vi "Do_channel_maths.vi"(4 "Output Index":i32, 5 "Channel Values In":string[][](array[string]), 6 "Channel Names":string[](array[string]), 7 "Maths Equation":string) -> (0 "Error String":string, 1 "Channel Values Out":string[][](array[string]))   [LabVIEW 2015]
uses:
  Data_plotting_vis/Results_plotter_Global.vi
  <vilib>/gmath/NI_Gmath.lvlib
panel:
  out "Generic Equation":string
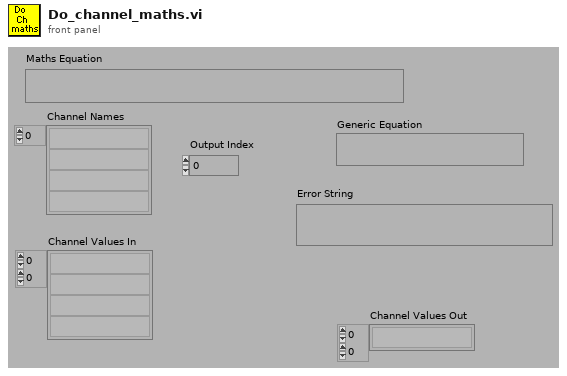
[diagram p1: front panel]
types:
  T1 = cluster{"Tables":i32[][], "Y Values":dbl[], "Variables input decode":i32[], i32[]}[]
  T2 = cluster{"Y Values":dbl[][], "Tables":i32[][][], "Variables input decode":i32[], "Variables output decode":i32[]}
  T3 = cluster{"Tables":i32[][], "Y Values":dbl[], "Variables input decode":i32[], i32[]}
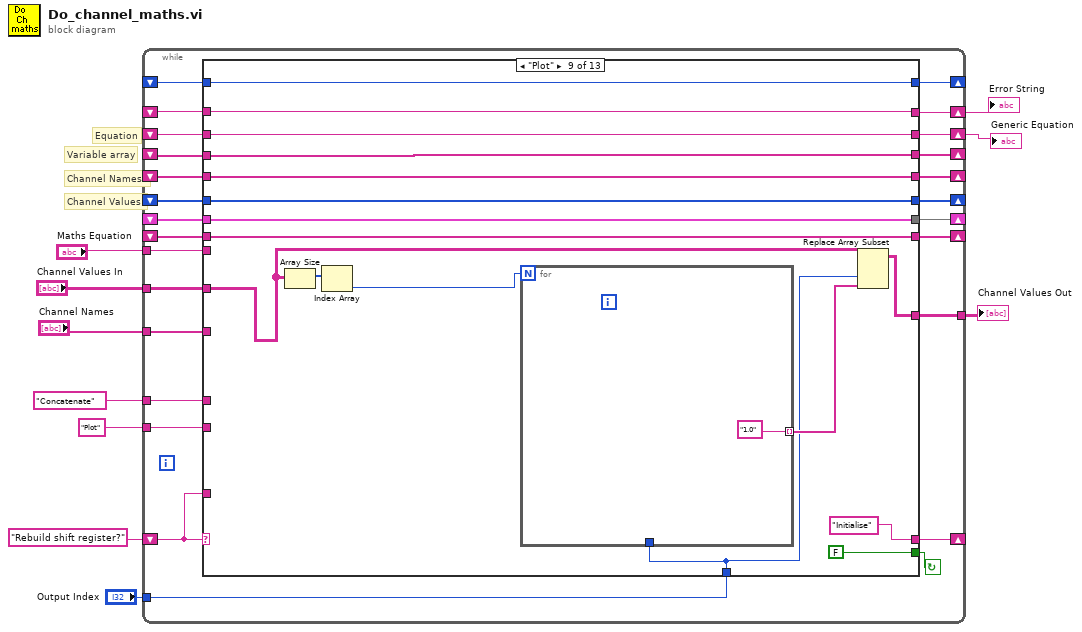
[diagram p0: block diagram]
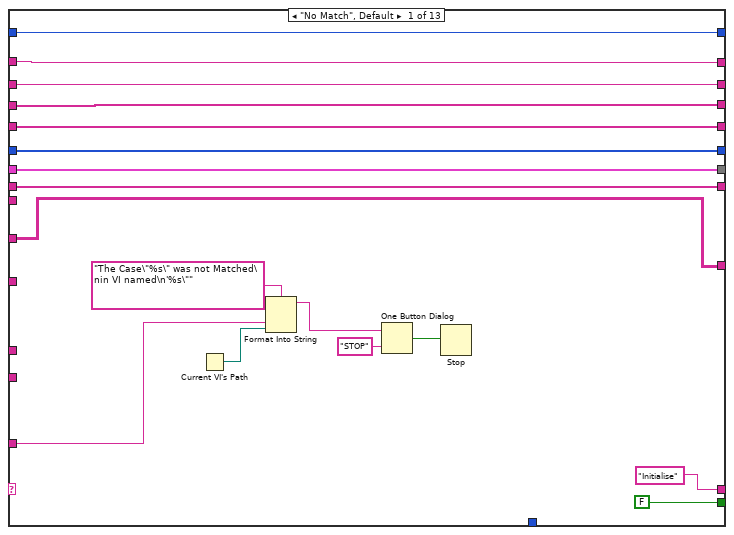
[diagram p2: hidden frame]
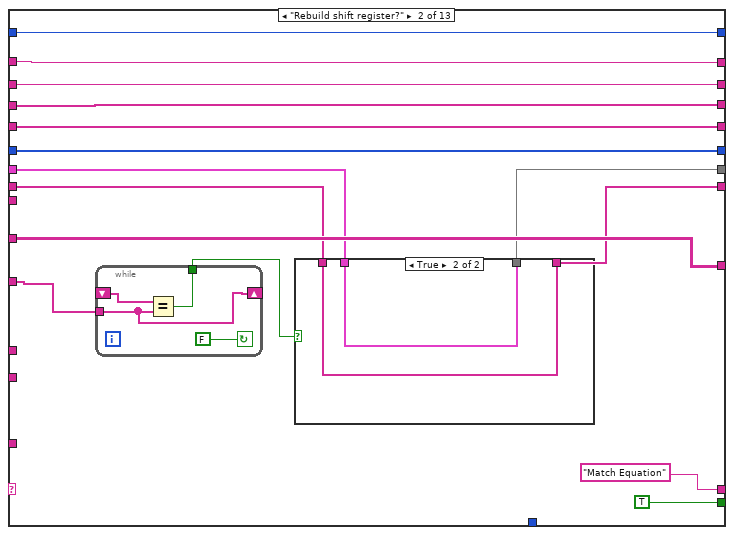
[diagram p3: hidden frame]
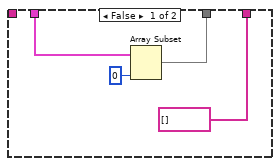
[diagram p4: hidden frame]
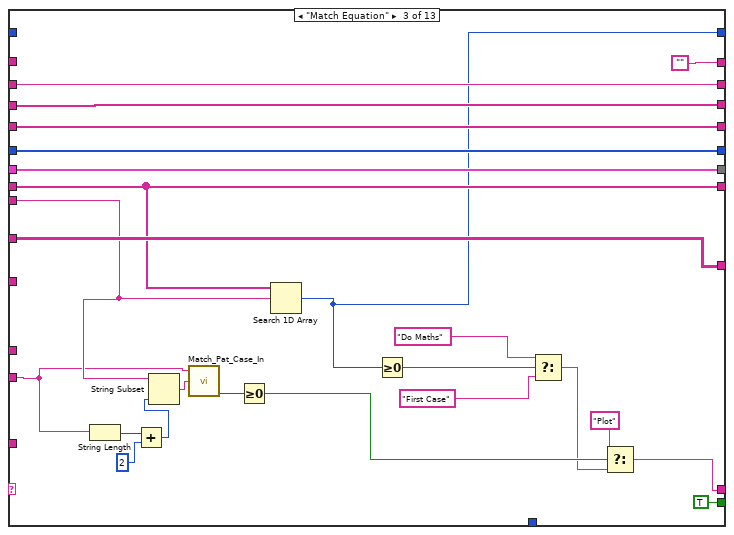
[diagram p5: hidden frame]
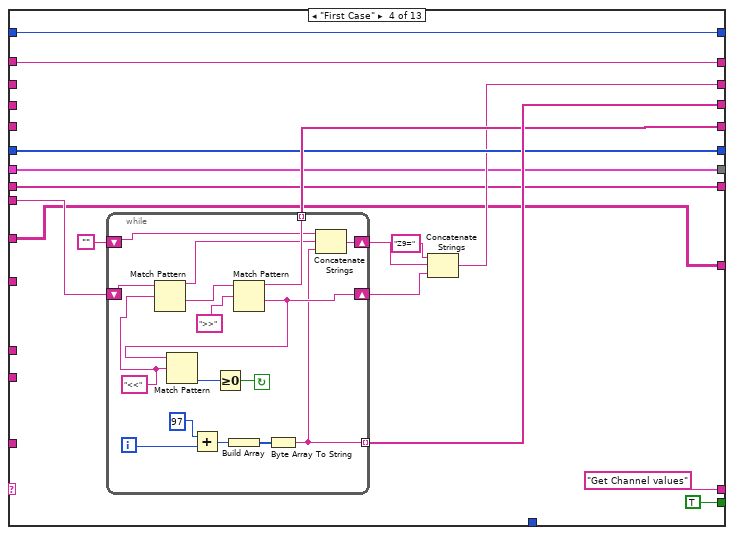
[diagram p6: hidden frame]
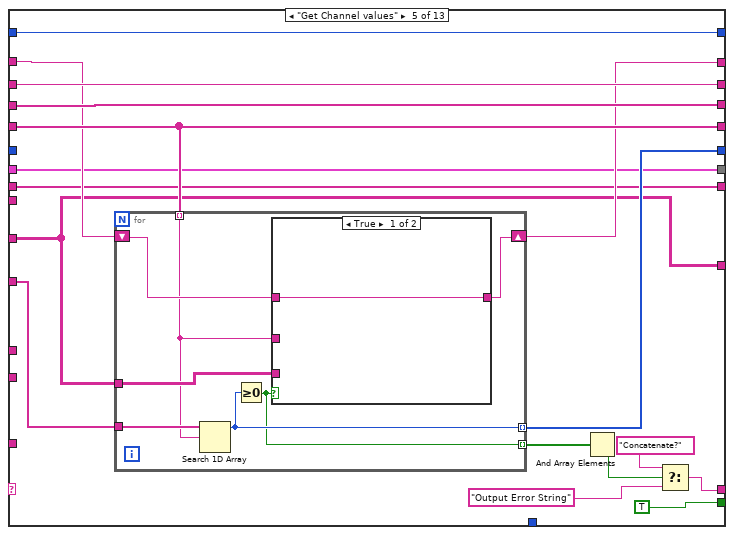
[diagram p7: hidden frame]
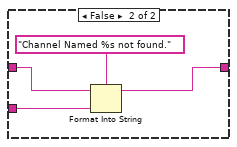
[diagram p8: hidden frame]
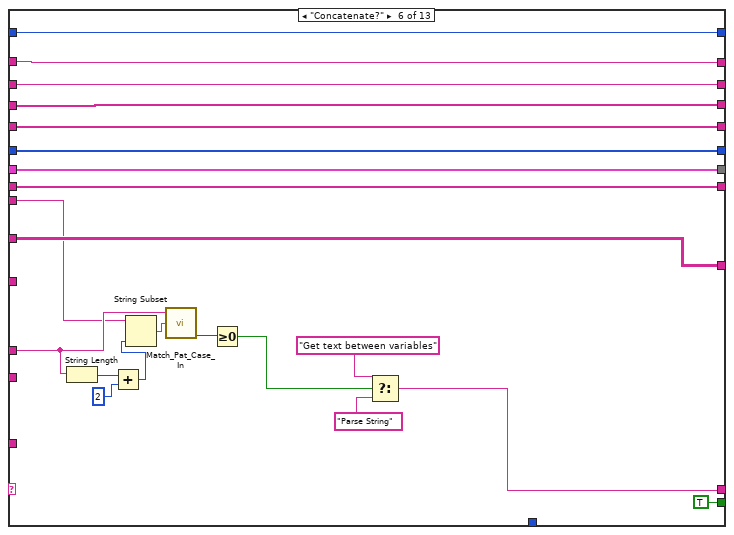
[diagram p9: hidden frame]
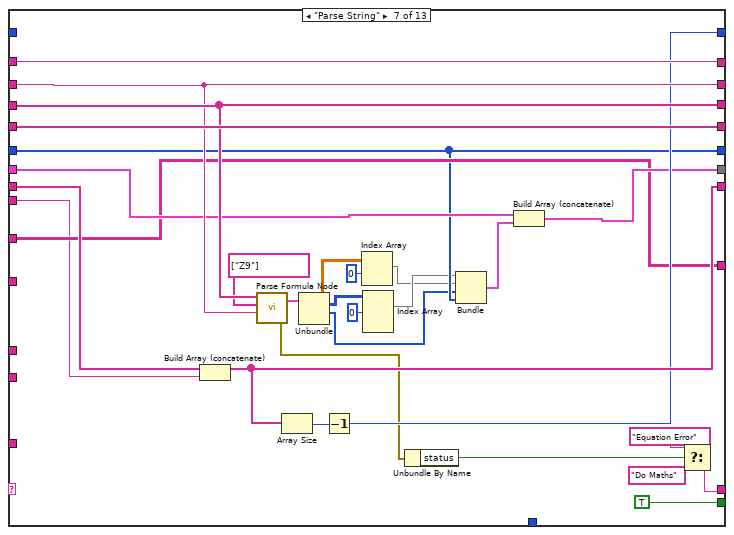
[diagram p10: hidden frame]
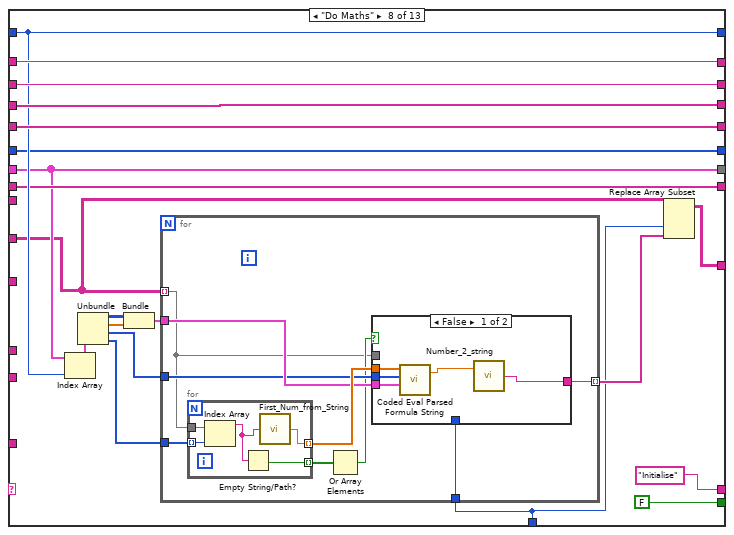
[diagram p11: hidden frame]
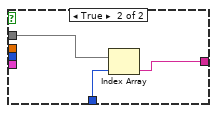
[diagram p12: hidden frame]
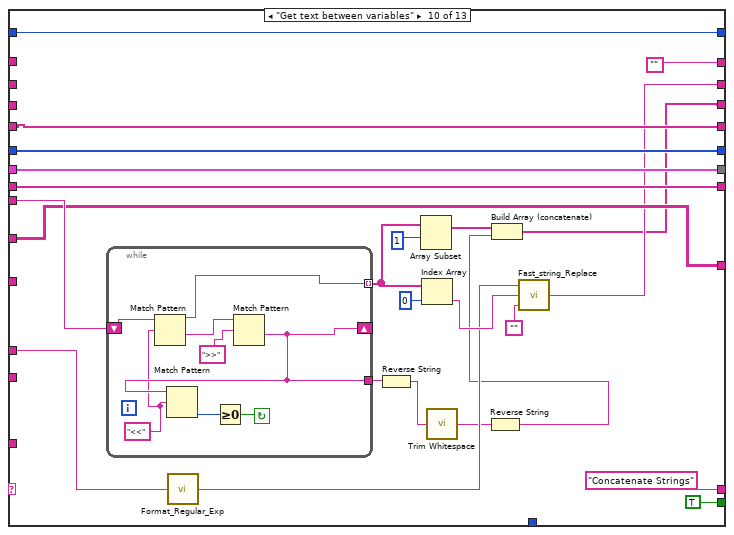
[diagram p13: hidden frame]
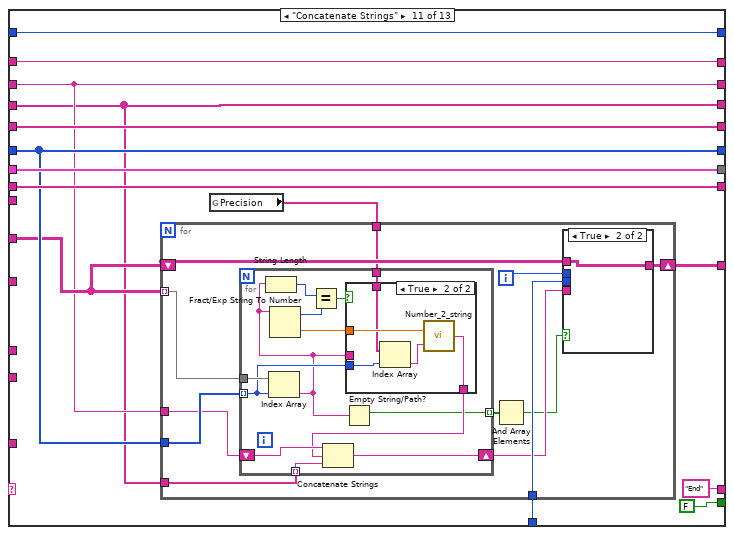
[diagram p14: hidden frame]
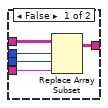
[diagram p15: hidden frame]
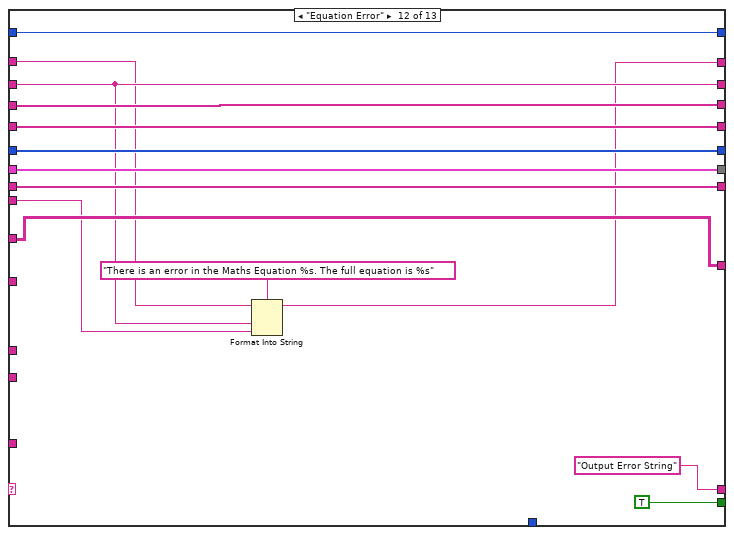
[diagram p17: hidden frame]
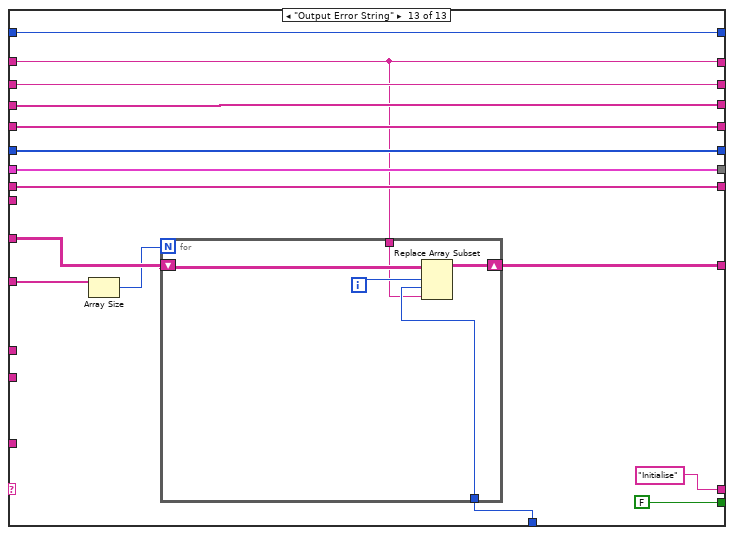
[diagram p18: hidden frame]
diagram:
  # "Channel Names"
  # "Variable array"
  # "Channel Values"
  # "Equation"
  n1 = while {
    tunnel: [w13] -> w4
    tunnel: "Output Index" -> [w14]
    shift-left: _ -> [w15]
    shift-right: [w16] -> _
    shift-left: _ -> [w19]
    shift-right: [w18] -> _
    shift-left: _ -> [w17]
    shift-right: [w20] -> _
    tunnel: "Channel Values In" -> [w21]
    tunnel: "Channel Names" -> [w22]
    tunnel: "Maths Equation" -> [w23]
    shift-left: _ -> [w25]
    shift-right: [w24] -> _
    shift-left: _ -> [w27]
    shift-right: [w26] -> _
    shift-left: _ -> [w29]
    shift-right: [w28] -> _
    shift-left: _ -> [w31]
    shift-right: [w30] -> w6
    shift-left: _ -> [w33]
    shift-right: [w32] -> w7
    shift-left: "Rebuild shift register?" -> [w34]
    shift-right: [w35] -> _
    tunnel: "Concatenate" ("regular expression") -> [w12]
    tunnel: "Plot" ("regular expression") -> [w11]
    stop <- w36 continue-if-true
    n2 = case shown="\"Plot\"" w34 {
      tunnel: [FALSE TRUE TRUE TRUE TRUE TRUE TRUE FALSE FALSE TRUE FALSE TRUE FALSE] -> w36
      tunnel: ["Initialise" "Match Equation" w80 "Get Channel values" w136 w173 w199 "Initialise" "Initialise" "Concatenate Strings" "End" "Output Error String" "Initialise"] -> w35
      tunnel: w34 -> [w48 _ _ _ _ _ _ _ _ _ _ _ _]
      tunnel: w33 -> [w45 w66 _ w103 w144 w184 w211 w230 w268 _ w315 w357 w370]
      tunnel: [w45 w66 "" w103 w145 w184 w211 w230 w268 "" w315 w356 w370] -> w32
      tunnel: w31 -> [w44 w65 w102 _ w150 w183 w207 w228 w266 _ w307 w359 w380]
      tunnel: [w44 w65 w102 w108 w150 w183 w207 w228 w266 w282 w307 w359 w380] -> w30
      tunnel: w29 -> [w43 w64 w101 _ w149 w182 w208 w229 w267 _ w306 w366 w381]
      tunnel: [w43 w64 w101 w115 w149 w182 w208 w229 w267 w277 w306 w366 w381] -> w28
      tunnel: w27 -> [w42 w63 w100 _ w147 w181 w212 w231 w269 w287 w316 w367 w382]
      tunnel: [w42 w63 w100 w111 w147 w181 w212 w231 w269 w287 w316 w367 w382] -> w26
      tunnel: w25 -> [w41 w62 w99 w110 _ w180 w198 w219 w262 w292 w311 w362 w374]
      tunnel: [w41 w62 w99 w110 w146 w180 w198 w219 w262 w292 w311 w362 w374] -> w24
      tunnel: w23 -> [_ _ w86 w116 _ w166 w185 _ _ w294 _ w358 _]
      tunnel: w22 -> [_ w59 _ _ w148 _ _ _ _ _ _ _ w372]
      tunnel: w21 -> [w37 w60 w97 w104 w140 w172 w203 w217 w258 w288 w310 w361 w373]
      tunnel: [w40 w57 w98 w107 w143 w179 w204 w225 w263 w291 w312 w363 w377] -> w20
      tunnel: w19 -> [w39 w55 w96 w106 w142 w178 w210 w226 w264 w290 w313 w364 w378]
      tunnel: [w39 w54 w96 w106 w142 w178 w209 w226 w264 w290 w313 w364 w378] -> w18
      tunnel: w17 -> [w40 w56 w98 w107 w143 w179 w206 w225 w263 w291 w312 w363 w377]
      tunnel: [w38 w61 w95 w105 w141 w177 w205 w227 w265 w289 w314 w365 w379] -> w16
      tunnel: w15 -> [w38 w61 _ w105 w141 w177 _ w227 w265 w289 w314 w365 w379]
      tunnel: w14 -> [_ _ _ _ _ _ _ w214 w259 _ w309 _ w376]
      tunnel: [w37 w60 w97 w104 w140 w172 w203 w216 w261 w288 w308 w361 w375] -> w13
      tunnel: w12 -> [_ _ _ _ _ w171 _ _ _ w284 _ _ _]
      tunnel: w11 -> [_ _ w85 _ _ _ _ _ _ _ _ _ _]
      frame "No Match", Default {
        n3 = Current VI's Path() -> (path=w47:path)
        n4 = Format Into String(format string="The Case\"%s\" was not Matched\nin VI named\n'%s\"" ("Format String"), w48, w47) -> (resulting string=w51:string)  [unwired: 2 in, 1 out]
        n5 = One Button Dialog(message=w51, button name ("OK")="STOP") -> (true=w49:bool)
        n6 = Stop(stop? (T)=w49) -> ()
      }
      frame "Rebuild shift register?" {
        n7 = while {
          shift-right: [w77] -> _
          shift-left: _ -> [w78]
          tunnel: w59 -> [w77]
          tunnel: [w76] -> w58
          stop <- FALSE continue-if-true
          n8 = Equal?(x=w78, y=w77) -> (x = y?=w76:bool)
        }
        n9 = case shown="True" w58 {
          tunnel: [w70 w74] -> w57
          tunnel: w56 -> [w72 w74]
          tunnel: w55 -> [_ w73]
          tunnel: [string[] [] w73] -> w54
          frame False {
            n10 = Array Subset(array=w72, length=0) -> (w70:T1)  [unwired: 1 in]
          }
          frame True {
          }
        }
      }
      frame "Match Equation" {
        n11 = String Length(string=w85) -> (length=w87:i32)
        n12 = Add(x=w87, y=2) -> (x+y=w89:i32)
        n13 = String Subset(string=w86, length (rest)=w89) -> (substring=w90:string)  [unwired: 1 in]
        n14 = call "Match_Pat_Case_In.vi"("String to match"=w85, "String"=w90) -> ("offset past match"=w83:i32)  [unwired: 1 in, 3 out]
        n15 = Greater Or Equal To 0?(x=w83) -> (x >= 0?=w82:bool)
        n16 = Search 1D Array(1D array=w96, element=w86) -> (index of element=w95:i32)  [unwired: 1 out]
        n17 = Greater Or Equal To 0?(x=w95) -> (x >= 0?=w94:bool)
        n18 = Select(t="Do Maths", s=w94, f="First Case") -> (s? t:f=w81:string)
        n19 = Select(t="Plot", s=w82, f=w81) -> (s? t:f=w80:string)
      }
      frame "First Case" {
        n20 = while {
          shift-left: "" -> [w121]
          shift-right: [w122] -> w113
          tunnel: [w123] -> w115 mode=indexing
          tunnel: [w129] -> w111 mode=indexing
          shift-left: w116 -> [w134]
          shift-right: [w132] -> w112
          i -> [w125]
          stop <- w130 continue-if-true
          w120 = "<<" ("regular expression")
          n21 = Match Pattern(string=w134, regular expression=w120) -> (before substring=w124:string, after substring=w133:string)  [unwired: 3 out]
          n22 = Add(x=97, y=w125) -> (x+y=w127:i32)
          n23 = Build Array(w127) -> (w128:i32[])
          n24 = Match Pattern(string=w133, regular expression=">>") -> (before substring=w129:string, after substring=w132:string)  [unwired: 3 out]
          n25 = Match Pattern(string=w132, regular expression=w120) -> (offset past match=w131:i32)  [unwired: 4 out]
          n26 = Greater Or Equal To 0?(x=w131) -> (x >= 0?=w130:bool)
          n27 = Byte Array To String(unsigned byte array=w128) -> (string=w123:string)
          n28 = Concatenate Strings(w121, w124, w123) -> (w122:string)
        }
        n29 = Concatenate Strings("Z9=" ("Substring"), w113, w112) -> (w108:string)
      }
      frame "Get Channel values" {
        n30 = for {
          tunnel: w148 -> [w158]
          tunnel: w147 -> [w154] mode=indexing
          tunnel: w140 -> [w157]
          tunnel: [w153] -> w146 mode=indexing
          shift-right: [w155] -> w145
          shift-left: w144 -> [w156]
          tunnel: [w152] -> w139 mode=indexing
          n31 = Search 1D Array(1D array=w158, element=w154) -> (index of element=w153:i32)  [unwired: 1 out]
          n32 = Greater Or Equal To 0?(x=w153) -> (x >= 0?=w152:bool)
          n33 = case shown="True" w152 {
            tunnel: w157 -> [_ _]
            tunnel: w154 -> [_ w163]
            tunnel: w156 -> [w159 w161]
            tunnel: [w159 w160] -> w155
            frame True {
            }
            frame False {
              n34 = Format Into String(format string="Channel Named %s not found." ("Format String"), initial string=w161, w163) -> (resulting string=w160:string)  [unwired: 1 in, 1 out]
            }
          }
        }
        n35 = And Array Elements(Boolean array=w139) -> (logical AND=w138:bool)
        n36 = Select(t="Concatenate?", s=w138, f="Output Error String") -> (s? t:f=w136:string)
      }
      frame "Concatenate?" {
        n37 = String Length(string=w171) -> (length=w170:i32)
        n38 = Add(x=w170, y=2) -> (x+y=w168:i32)
        n39 = String Subset(string=w166, length (rest)=w168) -> (substring=w167:string)  [unwired: 1 in]
        n40 = call "Match_Pat_Case_In.vi"("String to match"=w171, "String"=w167) -> ("offset past match"=w176:i32)  [unwired: 1 in, 3 out]
        n41 = Greater Or Equal To 0?(x=w176) -> (x >= 0?=w165:bool)
        n42 = Select(t="Get text between variables" ("regular expression"), s=w165, f="Parse String" ("regular expression")) -> (s? t:f=w173:string)
      }
      frame "Parse String" {
        n43 = Build Array (concatenate)(w210, w185) -> (w209:string[])
        n44 = call <vilib>:"Parse Formula Node.vi"("formula"=w207, "Variables Output"=string[] ["Z9"], "Variables Input"=w208) -> ("error out"=w186:errorcluster, "Parsed Formula Node"=w195:T2)  [unwired: 1 in]
        n45 = Array Size(array=w209) -> (size(s)=w196:i32)
        n46 = Unbundle(w195) -> ("Y Values"=w194:dbl[][], "Tables"=w191:i32[][][], "Variables input decode"=w188:i32[])  [unwired: 1 out]
        n47 = Decrement(x=w196) -> (x-1=w205:i32)
        n48 = Index Array(array=w194, index (row)=0 ("Index")) -> (element=w189:dbl[])  [unwired: 1 in]
        n49 = Index Array(array=w191, index (dim 0)=0 ("Index")) -> (element=w190:i32[][])  [unwired: 2 in]
        n50 = Unbundle By Name(w186) -> ("status"=w202:bool)
        n51 = Bundle("Tables"=w190, "Y Values"=w189, "Variables input decode"=w188, w198) -> (w187:T3)  [unwired: 1 out]
        n52 = Build Array (concatenate)(w206, w187) -> (w204:T1)
        n53 = Select(t="Equation Error", s=w202, f="Do Maths") -> (s? t:f=w199:string)
      }
      frame "Do Maths" {
        n54 = Index Array(array=w225, index=w227) -> (element=w224:T3)
        n55 = Unbundle(w224) -> ("Tables"=w223:i32[][], "Y Values"=w222:dbl[], "Variables input decode"=w220:i32[], w218:i32[])
        n56 = Bundle("Tables"=w223, "Y Values"=w222) -> (w221:cluster{"Tables":i32[][], "Y Values":dbl[]})  [unwired: 1 out]
        n57 = for {
          tunnel: w217 -> [w235] mode=indexing
          tunnel: w218 -> [w242]
          tunnel: w221 -> [w240]
          tunnel: w220 -> [w239]
          tunnel: [w236] -> w215 mode=indexing
          tunnel: w214 -> [w234]
          n58 = for {
            tunnel: w235 -> [w255]
            tunnel: w242 -> [w254] mode=indexing
            tunnel: [w251] -> w241 mode=indexing
            tunnel: [w253] -> w238 mode=indexing
            n59 = Index Array(array=w255, index=w254) -> (element=w252:string)
            n60 = Empty String/Path?(string/path=w252) -> (empty?=w253:bool)
            n61 = call "First_Num_from_String.vi"("string"=w252) -> ("number"=w251:dbl)
          }
          n62 = Or Array Elements(Boolean array=w238) -> (logical OR=w237:bool)
          n63 = case shown="False" w237 {
            tunnel: w241 -> [w247 _]
            tunnel: w240 -> [w246 _]
            tunnel: w239 -> [w245 _]
            tunnel: [w243 w248] -> w236
            tunnel: w235 -> [_ w250]
            tunnel: w234 -> [_ w249]
            frame False {
              n64 = call <vilib>:"Coded Eval Parsed Formula String.vi"("Parsed Formula"=w246, "Variables"=w245, "X Values"=w247) -> ("y value"=w244:dbl)  [unwired: 1 in, 1 out]
              n65 = call "Number_2_string.vi"("number"=w244) -> ("String"=w243:string)  [unwired: 1 in]
            }
            frame True {
              n66 = Index Array(array=w250, index=w249) -> (element=w248:string)
            }
          }
        }
        n67 = Replace Array Subset(array=w217, new element=w215, index (col)=w214) -> (w216:string[][])  [unwired: 1 in]
      }
      frame "Plot" {
        n68 = Array Size(array=w258) -> (size(s)=w257:i32[])
        n69 = Index Array(array=w257) -> (element=w256:i32)  [unwired: 1 in]
        n70 = for {
          N: w256 -> [_]
          tunnel: ["1.0"] -> w260 mode=indexing
          tunnel: w259 -> [_]
        }
        n71 = Replace Array Subset(array=w258, new element=w260, index (col)=w259) -> (w261:string[][])  [unwired: 1 in]
      }
      frame "Get text between variables" {
        n72 = while {
          shift-left: w294 -> [w304]
          shift-right: [w299] -> _
          tunnel: [w300] -> w280 mode=indexing
          tunnel: [w299] -> w276
          stop <- w301 continue-if-true
          w298 = "<<" ("regular expression")
          n73 = Match Pattern(string=w304, regular expression=w298) -> (before substring=w300:string, after substring=w303:string)  [unwired: 3 out]
          n74 = Match Pattern(string=w303, regular expression=">>") -> (after substring=w299:string)  [unwired: 4 out]
          n75 = Match Pattern(string=w299, regular expression=w298) -> (offset past match=w302:i32)  [unwired: 4 out]
          n76 = Greater Or Equal To 0?(x=w302) -> (x >= 0?=w301:bool)
        }
        n77 = call "Format_Regular_Exp.vi"("Regular expression"=w284) -> ("Case Insensitive for html"=w283:string)
        n78 = Reverse String(1:w276) -> (0:w275:string)
        n79 = Array Subset(array=w280, index=1) -> (w279:string[])  [unwired: 1 in]
        n80 = Index Array(array=w280, index=0) -> (element=w285:string)
        n81 = call <vilib>:"Trim Whitespace.vi"("string"=w275) -> ("trimmed string"=w274:string)  [unwired: 1 in]
        n82 = Reverse String(1:w274) -> (0:w273:string)
        n83 = Build Array (concatenate)(w279, w273) -> (w277:string[])
        n84 = call "Fast_string_Replace.vi"("Replace match with:"="", "Input String"=w285, "regular expression"=w283) -> ("Output String"=w282:string)  [unwired: 2 out]
      }
      frame "Concatenate Strings" {
        n85 = global read "Results_plotter_Global.vi" "Precision"() -> (w305:string[])
        n86 = for {
          tunnel: w310 -> [w330] mode=indexing
          shift-right: [w327] -> w308
          shift-left: w310 -> [w328]
          tunnel: w311 -> [w329]
          tunnel: w309 -> [w325]
          tunnel: w307 -> [w324]
          tunnel: w306 -> [w323]
          tunnel: w305 -> [w322]
          i -> [w326]
          n87 = for {
            tunnel: w330 -> [w349]
            tunnel: w329 -> [w341] mode=indexing
            shift-right: [w339] -> w321
            shift-left: w324 -> [w348]
            tunnel: w323 -> [w347] mode=indexing
            tunnel: w322 -> [w340]
            tunnel: [w337] -> w320 mode=indexing
            n88 = Index Array(array=w349, index=w341) -> (element=w338:string)
            n89 = String Length(string=w338) -> (length=w346:i32)
            n90 = Fract/Exp String To Number(string=w338) -> (offset past number=w345:i32, number=w343:dbl)  [unwired: 3 out]
            n91 = Equal?(x=w346, y=w345) -> (x = y?=w344:bool)
            n92 = Empty String/Path?(string/path=w338) -> (empty?=w337:bool)
            n93 = case shown="True" w344 {
              tunnel: w343 -> [_ w355]
              tunnel: [w350 w354] -> w342
              tunnel: w338 -> [w350 _]
              tunnel: w341 -> [_ w353]
              tunnel: w340 -> [_ w352]
              frame False {
              }
              frame True {
                n94 = Index Array(array=w352, index=w353) -> (element=w351:string)
                n95 = call "Number_2_string.vi"("precision"=w351, "number"=w355) -> ("String"=w354:string)
              }
            }
            n96 = Concatenate Strings(w348, w342, w347) -> (w339:string)
          }
          n97 = And Array Elements(Boolean array=w320) -> (logical AND=w319:bool)
          n98 = case shown="True" w319 {
            tunnel: w328 -> [w335 w336]
            tunnel: [w334 w336] -> w327
            tunnel: w326 -> [w333 _]
            tunnel: w325 -> [w332 _]
            tunnel: w321 -> [w331 _]
            frame False {
              n99 = Replace Array Subset(array=w335, new element=w331, index (row)=w333, index (col)=w332) -> (w334:string[][])
            }
            frame True {
            }
          }
        }
      }
      frame "Equation Error" {
        n100 = Format Into String(format string="There is an error in the Maths Equation %s. The full equation is %s", initial string=w357, w359, w358) -> (resulting string=w356:string)  [unwired: 1 in, 1 out]
      }
      frame "Output Error String" {
        n101 = Array Size(array=w372) -> (size(s)=w371:i32)
        n102 = for {
          N: w371 -> [_]
          shift-right: [w388] -> w375
          shift-left: w373 -> [w389]
          tunnel: w376 -> [w386]
          tunnel: w370 -> [w385]
          i -> [w387]
          n103 = Replace Array Subset(array=w389, new element=w385, index (row)=w387, index (col)=w386) -> (w388:string[][])
        }
      }
    }
  }
  "Error String" <- w7
  "Generic Equation" <- w6
  "Channel Values Out" <- w4
